vi "TB3000_frequency_set.vi"(8 "error in":errorcluster, 10 "Freq (MHz)":dbl=80.0, 11 "VISA resource name in":refnum<visa-resource-name>) -> (0 "error out":errorcluster, 3 "VISA resource name out":refnum<visa-resource-name>)   [LabVIEW 2021]
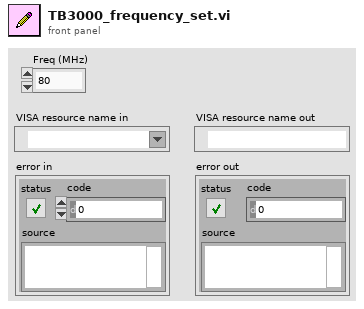
[diagram p1: front panel]
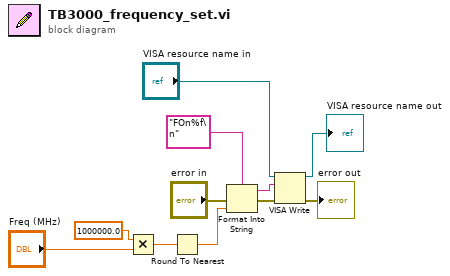
[diagram p0: block diagram]
diagram:
  n1 = Multiply(x=1000000.0, y="Freq (MHz)") -> (x*y=w4:dbl)
  n2 = Round To Nearest(number=w4) -> (nearest integer value=w3:dbl)
  n3 = Format Into String(format string="FOn%f\n", error in="error in", w3) -> (resulting string=w10:string, error out=w9:errorcluster)  [unwired: 1 in]
  n4 = VISA Write(VISA resource name="VISA resource name in", write buffer=w10, error in (no error)=w9) -> (VISA resource name out=→"VISA resource name out":refnum<visa-resource-name>, error out=→"error out":errorcluster)  [unwired: 1 out]
